vi "SubVI_Interpolate_EEG.vi"(8 "error in (no error)":errorcluster, 9 "Interpolant Size":dbl, 10 "Resampling rate":dbl, 11 "Converted EEG":T1) -> (0 "error out":errorcluster, 3 "EEG":T2)   [LabVIEW 2020]
uses:
  <extravilib>/ChannelInstances/Stream-a[.](dbl)/)Channel.ctl
  <extravilib>/ChannelInstances/Lossy Stream-a[.](dbl)/)Channel.ctl
  <extravilib>/ChannelInstances/Lossy Stream-a[.](dbl)/EndpointRead.vi
  <extravilib>/ChannelInstances/Stream-a[.](dbl)/Endpoint.vi
  Global 1.vi
  <extravilib>/ChannelInstances/Lossy Stream-a[.](dbl)/)Channel.vi
  <resource>/ChannelSupport/_ChannelSupport/WaitIfNeeded.vi
  <extravilib>/ChannelInstances/Stream-a[.](dbl)/)Channel.vi
  <vilib>/ptbypt/NI_PtbyPt.lvlib
  <extravilib>/ChannelInstances/Stream-a[.](dbl).lvlib
  <extravilib>/ChannelInstances/Lossy Stream-a[.](dbl).lvlib
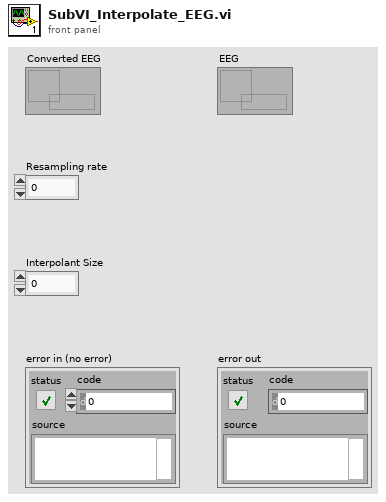
[diagram p1: front panel]
types:
  T1 = typedef "Lossy Stream-a[.](dbl).lvlib/)Channel.ctl" = refnum<queue>
  T2 = typedef "Stream-a[.](dbl).lvlib/)Channel.ctl" = refnum<queue>
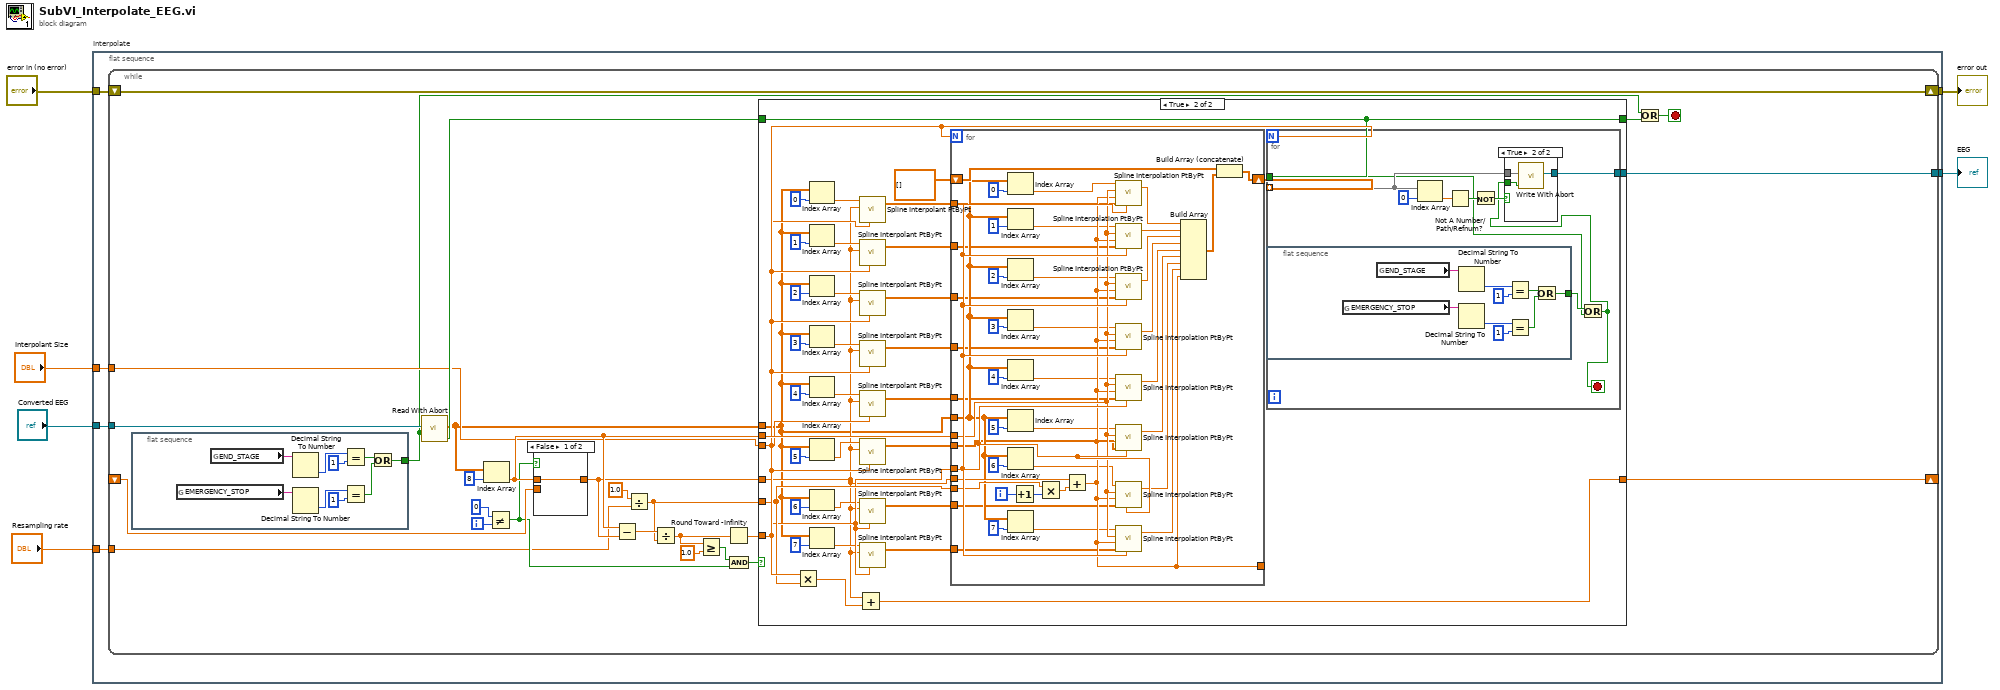
[diagram p0: block diagram]
diagram:
  n1 = flat-sequence "Interpolate" {
    tunnel: "Converted EEG" -> [w12]
    tunnel: [w11] -> w2
    tunnel: [w10] -> w3
    tunnel: "error in (no error)" -> [w9]
    tunnel: "Interpolant Size" -> [w8]
    tunnel: "Resampling rate" -> [w7]
    frame #0 {
      n2 = while {
        tunnel: w12 -> [w38]
        shift-right: [w23] -> _
        shift-left: _ -> [w29]
        tunnel: w8 -> [w24]
        tunnel: w7 -> [w14]
        tunnel: [w22] -> w11
        shift-right: [w20] -> w10
        shift-left: w9 -> [w20]
        i -> [w36]
        stop <- w18 stop-if-true
        n3 = flat-sequence {
          tunnel: [w39] -> w13
          frame #0 {
            n4 = global read "Global 1.vi" "EMERGENCY_STOP"() -> (w42:string)
            n5 = global read "Global 1.vi" "END_STAGE"() -> (w47:string)
            n6 = Decimal String To Number(string=w47) -> (number=w46:i32)  [unwired: 2 in, 1 out]
            n7 = Decimal String To Number(string=w42) -> (number=w44:i32)  [unwired: 2 in, 1 out]
            n8 = Equal?(x=w46, y=1) -> (x = y?=w40:bool)
            n9 = Equal?(x=w44, y=1) -> (x = y?=w41:bool)
            n10 = Or(x=w40, y=w41) -> (x .or. y?=w39:bool)
          }
        }
        n11 = call <extravilib>:"Read With Abort.vi"("abort"=w13, "channel"=w38) -> ("element"=w17:dbl[], "aborted?"=w25:bool)  [unwired: 3 in, 5 out]
        n12 = Index Array(array=w17, index=8 ("disabled index (col)")) -> (element=w28:dbl)
        n13 = Not Equal?(x=0, y=w36) -> (x != y?=w21:bool)
        n14 = case shown="False" w21 {
          tunnel: w29 -> [_ w49]
          tunnel: [w48 w49] -> w26
          tunnel: w28 -> [w48 _]
          frame False {
          }
          frame True {
          }
        }
        n15 = Subtract(x=w28, y=w26) -> (x-y=w33:dbl)
        n16 = Divide(x=1.0 ("Resampling rate"), y=w14) -> (x/y=w15:dbl)
        n17 = Divide(x=w33, y=w15) -> (x/y=w31:dbl)
        n18 = Greater Or Equal?(x=w31, y=1.0) -> (x >= y?=w35:bool)
        n19 = Round Toward -Infinity(1:w31) -> (0:w27:dbl)
        n20 = And(x=w35, y=w21) -> (x .and. y?=w30:bool)
        n21 = case shown="True" w30 {
          tunnel: w24 -> [_ w79]
          tunnel: w28 -> [_ w87]
          tunnel: w15 -> [_ w80]
          tunnel: w26 -> [w51 w54]
          tunnel: [w51 w85] -> w23
          tunnel: [_ w82] -> w22
          tunnel: w25 -> [w50 w52]
          tunnel: w27 -> [_ w81]
          tunnel: w17 -> [_ w53]
          tunnel: [w50 w52] -> w19
          frame False {
          }
          frame True {
            n22 = Multiply(x=w81, y=w80) -> (x*y=w86:dbl)
            n23 = Index Array(array=w53, index=0) -> (element=w55:dbl)
            n24 = Index Array(array=w53, index=1) -> (element=w56:dbl)
            n25 = Index Array(array=w53, index=2) -> (element=w57:dbl)
            n26 = Index Array(array=w53, index=3) -> (element=w58:dbl)
            n27 = Index Array(array=w53, index=4) -> (element=w59:dbl)
            n28 = Index Array(array=w53, index=5) -> (element=w60:dbl)
            n29 = Index Array(array=w53, index=6) -> (element=w61:dbl)
            n30 = Index Array(array=w53, index=7) -> (element=w62:dbl)
            n31 = Add(x=w54, y=w86) -> (x+y=w85:dbl)
            n32 = call <vilib>:"Spline Interpolant PtByPt.vi"("sample length"=w79, "x"=w54, "y"=w55) -> ("Interpolant"=w71:dbl[])  [unwired: 3 in, 1 out]
            n33 = call <vilib>:"Spline Interpolant PtByPt.vi"("sample length"=w79, "x"=w54, "y"=w56) -> ("Interpolant"=w72:dbl[])  [unwired: 3 in, 1 out]
            n34 = call <vilib>:"Spline Interpolant PtByPt.vi"("sample length"=w79, "x"=w54, "y"=w57) -> ("Interpolant"=w73:dbl[])  [unwired: 3 in, 1 out]
            n35 = call <vilib>:"Spline Interpolant PtByPt.vi"("sample length"=w79, "x"=w54, "y"=w58) -> ("Interpolant"=w74:dbl[])  [unwired: 3 in, 1 out]
            n36 = call <vilib>:"Spline Interpolant PtByPt.vi"("sample length"=w79, "x"=w54, "y"=w59) -> ("Interpolant"=w75:dbl[])  [unwired: 3 in, 1 out]
            n37 = call <vilib>:"Spline Interpolant PtByPt.vi"("sample length"=w79, "x"=w54, "y"=w60) -> ("Interpolant"=w76:dbl[])  [unwired: 3 in, 1 out]
            n38 = call <vilib>:"Spline Interpolant PtByPt.vi"("sample length"=w79, "x"=w54, "y"=w61) -> ("Interpolant"=w77:dbl[])  [unwired: 3 in, 1 out]
            n39 = call <vilib>:"Spline Interpolant PtByPt.vi"("sample length"=w79, "x"=w54, "y"=w62) -> ("Interpolant"=w78:dbl[])  [unwired: 3 in, 1 out]
            n40 = for {
              N: w81 -> [_]
              tunnel: w79 -> [w152]
              tunnel: w71 -> [w116]
              tunnel: w72 -> [w115]
              tunnel: w73 -> [w114]
              tunnel: w74 -> [w113]
              tunnel: w75 -> [w112]
              tunnel: w76 -> [w111]
              tunnel: w77 -> [w110]
              tunnel: w78 -> [w109]
              tunnel: w87 -> [w144]
              tunnel: w80 -> [w140]
              tunnel: w54 -> [w143]
              tunnel: [w142] -> _
              shift-right: [w138] -> w83
              shift-left: dbl[][] [] -> [w137]
              tunnel: w53 -> [w117]
              i -> [w120]
              n41 = Index Array(array=w117, index=0) -> (element=w128:dbl)
              n42 = Index Array(array=w117, index=1) -> (element=w127:dbl)
              n43 = Index Array(array=w117, index=2) -> (element=w126:dbl)
              n44 = Index Array(array=w117, index=3) -> (element=w125:dbl)
              n45 = Index Array(array=w117, index=4) -> (element=w124:dbl)
              n46 = Index Array(array=w117, index=5) -> (element=w123:dbl)
              n47 = Index Array(array=w117, index=6) -> (element=w122:dbl)
              n48 = Index Array(array=w117, index=7) -> (element=w121:dbl)
              n49 = Increment(x=w120) -> (x+1=w119:i32)
              n50 = Multiply(x=w140, y=w119) -> (x*y=w139:dbl)
              n51 = Add(x=w143, y=w139) -> (x+y=w142:dbl)
              n52 = call <vilib>:"Spline Interpolation PtByPt.vi"("sample length"=w152, "Interpolant"=w116, "x value"=w142, "x"=w144, "y"=w128) -> ("interpolation value"=w141:dbl)  [unwired: 1 in, 1 out]
              n53 = call <vilib>:"Spline Interpolation PtByPt.vi"("sample length"=w152, "Interpolant"=w115, "x value"=w142, "x"=w144, "y"=w127) -> ("interpolation value"=w151:dbl)  [unwired: 1 in, 1 out]
              n54 = call <vilib>:"Spline Interpolation PtByPt.vi"("sample length"=w152, "Interpolant"=w114, "x value"=w142, "x"=w144, "y"=w126) -> ("interpolation value"=w150:dbl)  [unwired: 1 in, 1 out]
              n55 = call <vilib>:"Spline Interpolation PtByPt.vi"("sample length"=w152, "Interpolant"=w113, "x value"=w142, "x"=w144, "y"=w125) -> ("interpolation value"=w149:dbl)  [unwired: 1 in, 1 out]
              n56 = call <vilib>:"Spline Interpolation PtByPt.vi"("sample length"=w152, "Interpolant"=w112, "x value"=w142, "x"=w144, "y"=w124) -> ("interpolation value"=w148:dbl)  [unwired: 1 in, 1 out]
              n57 = call <vilib>:"Spline Interpolation PtByPt.vi"("sample length"=w152, "Interpolant"=w111, "x value"=w142, "x"=w144, "y"=w123) -> ("interpolation value"=w147:dbl)  [unwired: 1 in, 1 out]
              n58 = call <vilib>:"Spline Interpolation PtByPt.vi"("sample length"=w152, "Interpolant"=w110, "x value"=w142, "x"=w144, "y"=w122) -> ("interpolation value"=w146:dbl)  [unwired: 1 in, 1 out]
              n59 = call <vilib>:"Spline Interpolation PtByPt.vi"("sample length"=w152, "Interpolant"=w109, "x value"=w142, "x"=w144, "y"=w121) -> ("interpolation value"=w145:dbl)  [unwired: 1 in, 1 out]
              n60 = Build Array(w141, w151, w150, w149, w148, w147, w146, w145, w142) -> (w118:dbl[])
              n61 = Build Array (concatenate)(w137, w118) -> (w138:dbl[][])
            }
            n62 = for {
              N: w81 -> [_]
              tunnel: w83 -> [w93] mode=indexing
              tunnel: w52 -> [w89]
              tunnel: [w96] -> w82
              stop <- w88 stop-if-true
              n63 = flat-sequence {
                tunnel: [w97] -> w90
                frame #0 {
                  n64 = global read "Global 1.vi" "EMERGENCY_STOP"() -> (w100:string)
                  n65 = global read "Global 1.vi" "END_STAGE"() -> (w105:string)
                  n66 = Decimal String To Number(string=w105) -> (number=w104:i32)  [unwired: 2 in, 1 out]
                  n67 = Decimal String To Number(string=w100) -> (number=w102:i32)  [unwired: 2 in, 1 out]
                  n68 = Equal?(x=w104, y=1) -> (x = y?=w98:bool)
                  n69 = Equal?(x=w102, y=1) -> (x = y?=w99:bool)
                  n70 = Or(x=w98, y=w99) -> (x .or. y?=w97:bool)
                }
              }
              n71 = Index Array(array=w93, index=0) -> (element=w94:dbl)
              n72 = Not A Number/Path/Refnum?(number/path/refnum=w94) -> (NaN/Path/Refnum?=w92:bool)
              n73 = Not(x=w92) -> (.not. x?=w91:bool)
              n74 = Or(x=w90, y=w89) -> (x .or. y?=w88:bool)
              n75 = case shown="True" w91 {
                tunnel: w88 -> [_ w107]
                tunnel: [_ w106] -> w96
                tunnel: w93 -> [_ w108]
                frame False {
                }
                frame True {
                  n76 = call <extravilib>:"Write With Abort.vi"("abort"=w107, "element"=w108) -> ("channel"=w106:T2)  [unwired: 6 in, 3 out]
                }
              }
            }
          }
        }
        n77 = Or(x=w13, y=w19) -> (x .or. y?=w18:bool)
      }
    }
  }
  "error out" <- w3
  "EEG" <- w2
